vi "detector_set_integration_time_seconds.vi"(8 "error in (no error)":errorcluster, 10 "integration time (seconds)":dbl, 11 "picoharp in":refnum<class "picoharp.lvclass">) -> (0 "error out":errorcluster, 3 "picoharp out":refnum<class "picoharp.lvclass">)   [LabVIEW 2015, in "picoharp.lvclass"]
uses:
  picoharp.lvclass
  picoharp.lvclass/picoharp.ctl
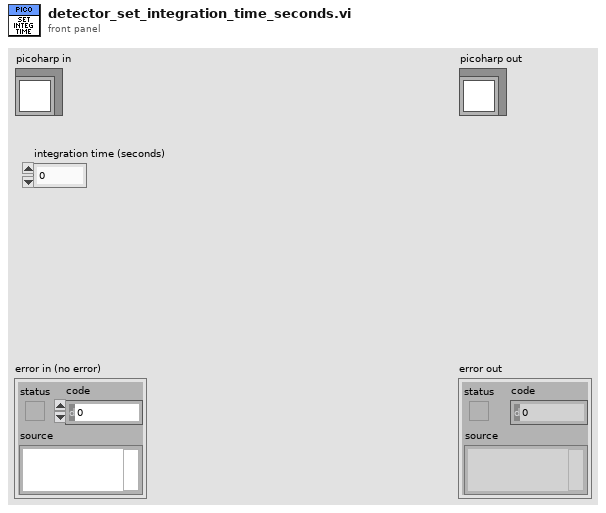
[diagram p1: front panel]
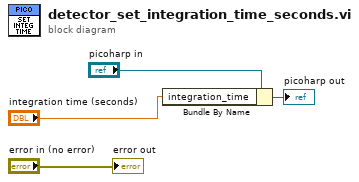
[diagram p0: block diagram]
diagram:
  n1 = Bundle By Name(cluster="picoharp in", "integration_time"="integration time (seconds)") -> (→"picoharp out":refnum<class "picoharp.lvclass">)
  "error out" <- "error in (no error)"
